vi "Pre Launch Init.vi"(11 "Nested in":refnum<class "Manager.lvclass">) -> (0 "error out":errorcluster, 3 "Nested out":refnum<class "Manager.lvclass">)   [LabVIEW 2025, in "Manager.lvlib" / "Manager.lvclass"]
doc: "(<B>Filename</B>: Actor Framework.lvlib:Actor.lvclass:Pre Launch Init.vi)\n\nDefines behavior that occurs after the Launch Nested Actor method is invoked but before the actor's Actor Core method begins running.\n\nBy default, this method does nothing. A descendant class may override it to define behavior."
uses:
  Manager.lvclass
  Manager.lvclass/Manager.ctl
  <vilib>/ActorFramework/Actor/Actor.lvclass
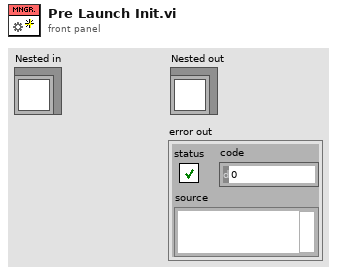
[diagram p1: front panel]
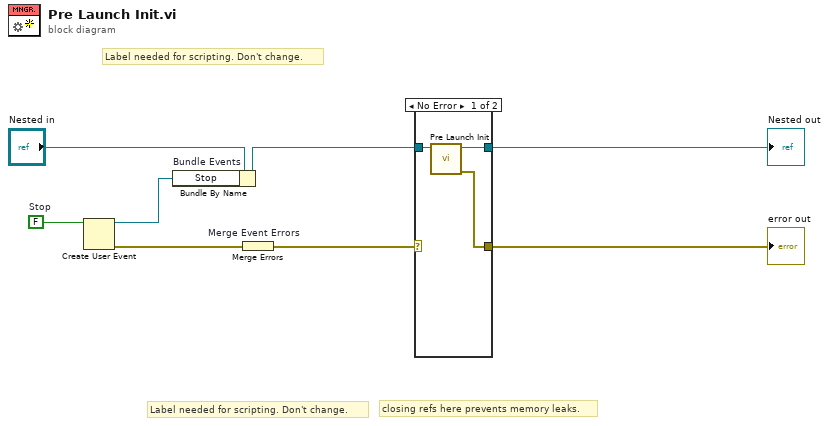
[diagram p0: block diagram]
diagram:
  w7 = FALSE  # Stop
  # "Label needed for scripting. Don't change."
  # "Label needed for scripting. Don't change."
  # "closing refs here prevents memory leaks."
  n1 = Create User Event(user event datatype=w7) -> (user event=w5:refnum<user-event>, error out=w6:errorcluster)  [unwired: 1 in]
  n2 = Bundle By Name "Bundle Events"(cluster="Nested in", "Stop"=w5) -> (w4:refnum<class "Manager.lvclass">)
  n3 = Merge Errors "Merge Event Errors"(w6) -> (w3:errorcluster)
  n4 = case shown="No Error" w3 {
    selector: w3 -> [_ w13]
    tunnel: [w11 w12] -> w2
    tunnel: w4 -> [w10 w12]
    tunnel: [w9 w13] -> w1
    frame No Error {
      n5 = call-parent "Pre Launch Init.vi"("Actor in"=w10) -> ("error out"=w9:errorcluster, "Actor out"=w11:refnum<class "Manager.lvclass">)  [unwired: 9 in]
    }
    frame Error {
    }
  }
  "error out" <- w1
  "Nested out" <- w2
